vi "PLL -- data source -- V3 -- meta.vi"(6 "set-get delay (msec)":i64, 7 "data source action":T2=enum."get", 9 "z  in (V)":cdb, 10 "Freq in (Hz)":dbl=40000.0 format="%#_13g", 11 "PLL data source":T1=enum."MFLI") -> (1 "z out (V)":cdb=0.00010527635459-2.9308681405e-05i, 2 "Freq out (Hz)":dbl=55115.2, 3 "PLL data source OUT":T1=enum."MFLI")   [LabVIEW 2018]
uses:
  publisher action.ctl
  PLL data source.ctl
  data source action.ctl
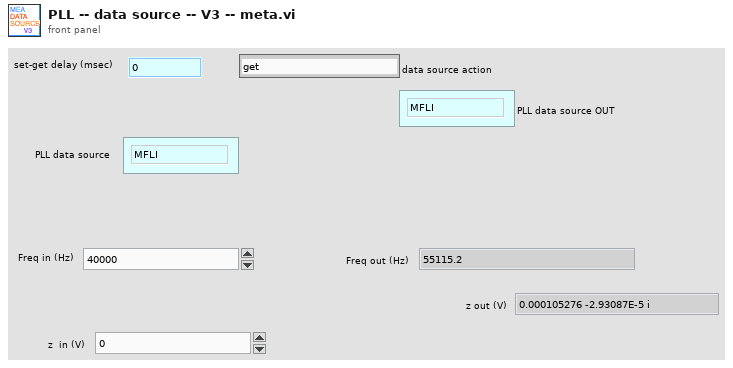
[diagram p1: front panel]
types:
  T1 = typedef "PLL data source.ctl" = enum16{"meta", "MFLI", "SRS865A", "arydh"}
  T2 = typedef "data source action.ctl" = enum16{"set", "get", "init", "set-and-get", "init source"}
  T3 = typedef "publisher action.ctl" = enum16{"set", "get", "init", "check"}
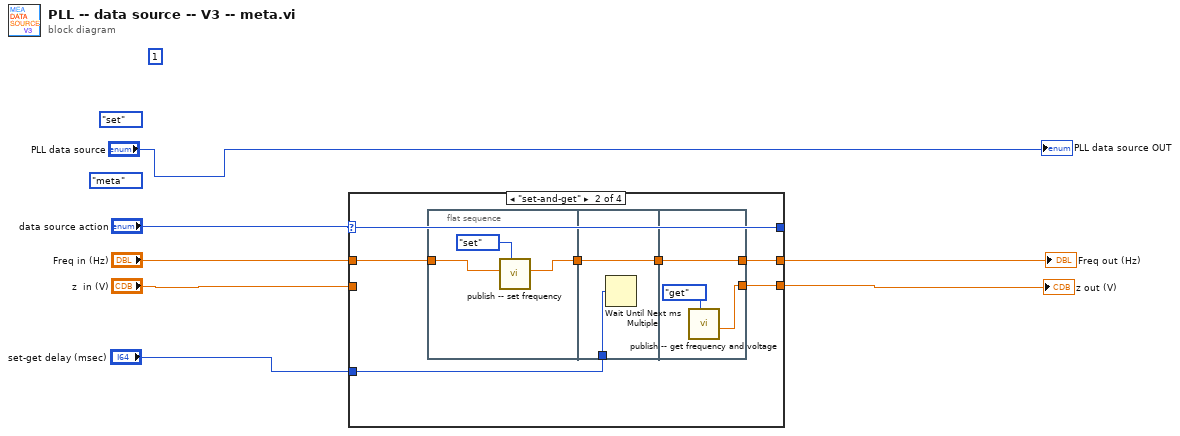
[diagram p0: block diagram]
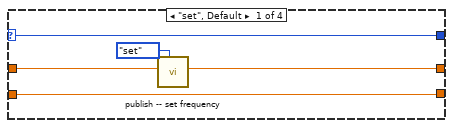
[diagram p2: hidden frame]
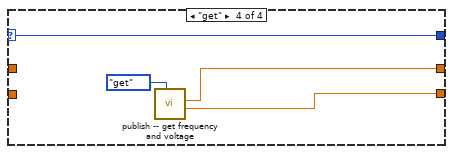
[diagram p4: hidden frame]
diagram:
  (unwired) 1
  (unwired) data_source_action."set" ("data source action")
  (unwired) PLL_data_source."meta" ("PLL data source")
  n1 = case shown="\"set-and-get\"" "data source action" {
    selector: "data source action" -> [w9 w17 w29 w32]
    tunnel: [w10 w18 w30 w33] -> w6
    tunnel: "Freq in (Hz)" -> [w11 w19 w30 _]
    tunnel: [w9 w17 w29 w32] -> _
    tunnel: "set-get delay (msec)" -> [_ w14 _ _]
    tunnel: [w8 w13 w28 w31] -> w2
    tunnel: "z  in (V)" -> [w8 _ w28 _]
    frame "set", Default {
      n2 = call "publish -- set frequency.vi"("publisher action"=publisher_action."set", "freq IN (Hz)"=w11) -> ("freq out (Hz)"=w10:dbl)  [unwired: 9 in]
    }
    frame "set-and-get" {
      n3 = flat-sequence {
        tunnel: w19 -> [w21]
        tunnel: [w20] -> w16
        tunnel: w16 -> [w24]
        tunnel: [w24] -> w15
        tunnel: w14 -> [w23]
        tunnel: [w27] -> w18
        tunnel: w15 -> [w27]
        tunnel: [w25] -> w13
        frame #0 {
          n4 = call "publish -- set frequency.vi"("publisher action"=publisher_action."set", "freq IN (Hz)"=w21) -> ("freq out (Hz)"=w20:dbl)  [unwired: 9 in]
        }
        frame #1 {
          n5 = Wait Until Next ms Multiple(millisecond multiple=w23) -> ()  [unwired: 1 out]
        }
        frame #2 {
          n6 = call "publish -- get frequency and voltage.vi"("publisher action"=publisher_action."get") -> ("Voltage out (V)"=w25:cdb)  [unwired: 8 in, 2 out]
        }
      }
    }
    frame "init" {
    }
    frame "get" {
      n7 = call "publish -- get frequency and voltage.vi"("publisher action"=publisher_action."get") -> ("Voltage out (V)"=w31:cdb, "freq out (Hz)"=w33:dbl)  [unwired: 8 in, 1 out]
    }
  }
  "Freq out (Hz)" <- w6
  "z out (V)" <- w2
  "PLL data source OUT" <- "PLL data source"
